vi "Read.vi"(8 "error in (no error)":errorcluster, 11 "Add in":refnum<class "AbsComp_Two Term_I64.lvclass">) -> (0 "error out":errorcluster, 2 "Result":bool, 3 "Add out":refnum<class "AbsComp_Two Term_I64.lvclass">)   [LabVIEW 2021, in "AbsComp_Two Term_I64.lvclass"]
uses:
  AbsComp_Two Term_I64.lvclass
  AbsComp_Two Term_I64.lvclass/AbsComp_Two Term_I64.ctl
  Abs_Types/I64 Integer/Abs_I64 Integer.lvclass
  Abs_Types/Numeric/Abs_Numeric.lvclass
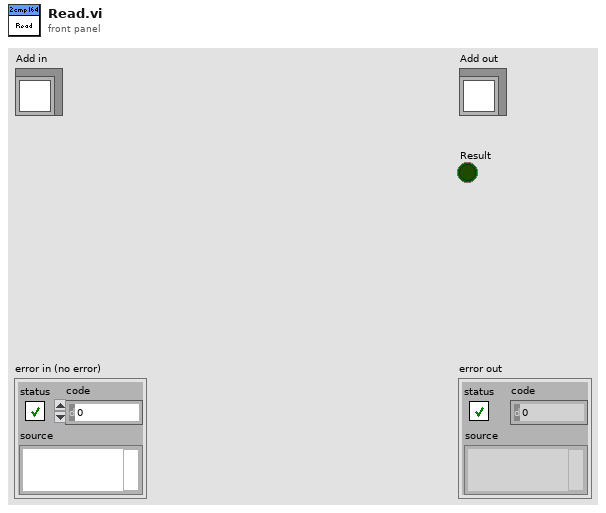
[diagram p1: front panel]
types:
  T1 = typedef "AbsComp_Two Term_I64.lvclass/Abstract Type.ctl" = refnum<class "Abs_I64 Integer.lvclass">
  T2 = typedef "Abs_I64 Integer.lvclass/Type.ctl" = i64
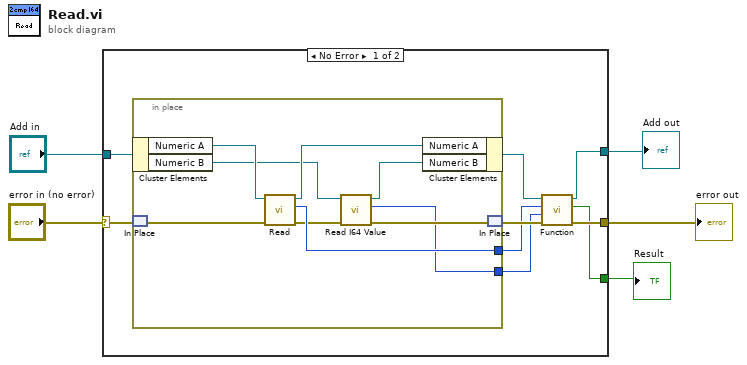
[diagram p0: block diagram]
diagram:
  n1 = case shown="No Error" "error in (no error)" {
    selector: "error in (no error)" -> [w13 w24]
    tunnel: "Add in" -> [w14 w25]
    tunnel: [w10 w25] -> w3
    tunnel: [w9 w24] -> w2
    tunnel: [w6 _] -> w1
    frame No Error {
      n2 = in-place {
        in-place-border: [w20] -> w8
        in-place-border: [w15] -> w7
        n3 = in-place-cluster #1(w14) -> ("Numeric A"=w23:T1, "Numeric B"=w19:refnum<class "Abs_Numeric.lvclass">)
        n4 = in-place-match #2(w13) -> (w22:errorcluster)
        n5 = call-dynamic "Read.vi"("error in (no error)"=w22, "Double Float.lvclass_340760 in"=w23) -> ("error out"=w17:errorcluster, "Value"=w20:T2, "Double Float.lvclass_340760 out"=w21:T1)  [unwired: 7 in]
        n6 = call-dynamic "Read I64 Value.vi"("error in (no error)"=w17, "Numeric in"=w19) -> ("error out"=w16:errorcluster, "I64 Value"=w15:i64, "Numeric out"=w18:refnum<class "Abs_Numeric.lvclass">)  [unwired: 7 in]
        n7 = in-place-cluster #1("Numeric A"=w21, "Numeric B"=w18) -> (w11:refnum<class "AbsComp_Two Term_I64.lvclass">)
        n8 = in-place-match #2(w16) -> (w12:errorcluster)
      }
      n9 = call-dynamic "Function.vi"("error in (no error)"=w12, "Numeric B"=w7, "Numeric A"=w8, "Two Terminal in"=w11) -> ("error out"=w9:errorcluster, "Result"=w6:bool, "Two Terminal out"=w10:refnum<class "AbsComp_Two Term_I64.lvclass">)  [unwired: 5 in]
    }
    frame Error {
    }
  }
  "error out" <- w2
  "Add out" <- w3
  "Result" <- w1
